vi "LogEvent.vi"(7 "Event Level":T1, 8 "error in (no error)":errorcluster, 9 "Data To Log":string, 10 "SourceID":string, 11 "Logger in":refnum<class "Logger.lvclass">) -> (0 "error out":errorcluster, 3 "Logger out":refnum<class "Logger.lvclass">)   [LabVIEW 2020, in "Event Log.lvlib" / "Logger.lvclass"]
uses:
  Logger.lvclass
  <vilib>/gpm_packages/@cs/event-logger/Source/Composed Log/Types/Log Level.ctl
  Logger.lvclass/Logger.ctl
  <vilib>/gpm_packages/@cs/event-logger/Source/Composed Log/LoggerReference/LoggerReference.lvclass/LoggerReference.ctl
  <vilib>/gpm_packages/@cs/event-logger/Source/Composed Log/LoggerReference/Log.vi
  <vilib>/gpm_packages/@cs/event-logger/Source/Composed Log/LoggerReference/Get Valid Event Time.vi
  <vilib>/gpm_packages/@cs/event-logger/Source/Composed Log/LoggerReference/Remove Stale Logs.vi
  <vilib>/gpm_packages/@cs/event-logger/Source/Composed Log/LoggerReference/LoggerReference.lvclass
  <vilib>/gpm_packages/@cs/event-logger/Source/Composed Log/Composed Log.lvlib
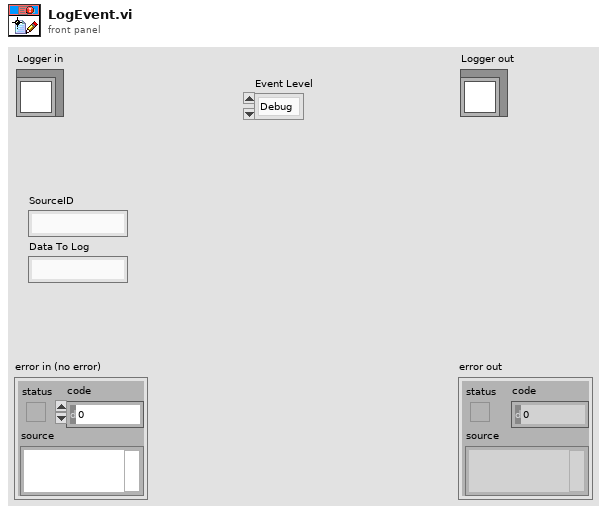
[diagram p1: front panel]
types:
  T1 = typedef "Composed Log.lvlib/Log Level.ctl" = enum16{"Debug", "Info", "Warning", "Error", "Critical"}
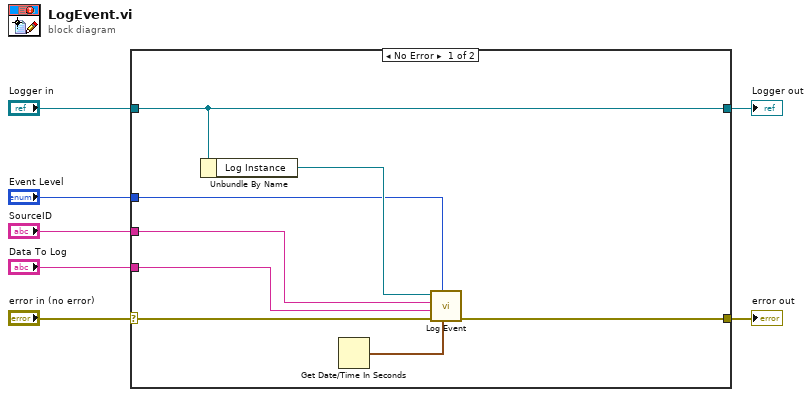
[diagram p0: block diagram]
diagram:
  n1 = case shown="No Error" "error in (no error)" {
    selector: "error in (no error)" -> [w13 w17]
    tunnel: [w12 w17] -> w6
    tunnel: [w15 w16] -> w4
    tunnel: "Logger in" -> [w15 w16]
    tunnel: "Event Level" -> [w11 _]
    tunnel: "SourceID" -> [w10 _]
    tunnel: "Data To Log" -> [w9 _]
    frame No Error {
      n2 = Unbundle By Name(w15) -> ("Log Instance"=w14:refnum<class "LoggerReference.lvclass">)
      n3 = Get Date/Time In Seconds() -> (seconds since 1Jan1904=w8:timestamp)
      n4 = call <vilib>:"Log Event.vi"("Event Time"=w8, "Event Level"=w11, "error in (no error)"=w13, "Data To Log"=w9, "SourceID"=w10, "Log Instance"=w14) -> ("error out"=w12:errorcluster)  [unwired: 4 in, 1 out]
    }
    frame Error {
    }
  }
  "error out" <- w6
  "Logger out" <- w4
